vi "disconnect.vi"(8 "error in (no error)":errorcluster, 11 "ID In":i32) -> (0 "error out":errorcluster)   [LabVIEW 2022 SP3, in "EClib functions.lvlib"]
doc: "This VI closes the IP connection between the computer and the instrument."
uses:
  EClib functions.lvlib
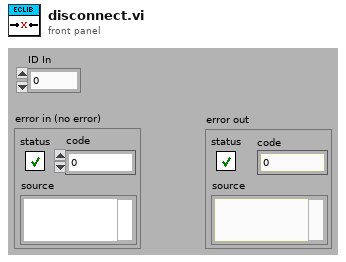
[diagram p1: front panel]
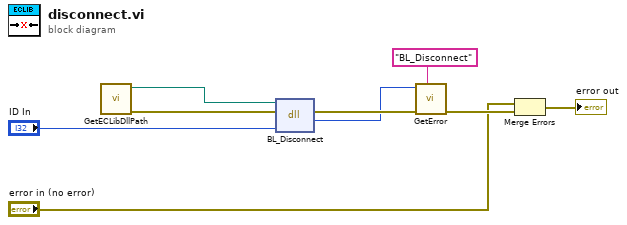
[diagram p0: block diagram]
diagram:
  n1 = call "GetECLibDllPath.vi"() -> ("error out"=w4:errorcluster, "ECLibDLLPath"=w8:path)  [unwired: 10 in]
  n2 = dll-call lib="?" fn="BL_Disconnect"(path in=w8, error in=w4, "arg1"="ID In") -> (error out=w7:errorcluster, "return type"=w1:i32)  [unwired: 2 in, 1 out]
  n3 = call "GetError.vi"("DLLFunction"="BL_Disconnect", "error in"=w7, "code"=w1) -> ("error out"=w6:errorcluster)  [unwired: 8 in]
  n4 = Merge Errors("error in (no error)", w6) -> (→"error out":errorcluster)
